vi "add to flattened hierarchy.vi"(8 "error in":errorcluster, 9 "instance data in":T1, 10 "parent ID":string, 11 "flattened hierarchy in":T2) -> (0 "error out":errorcluster, 3 "flattened hierarchy out":T2)   [LabVIEW 2013, in "NISE_CEF_TreeSerializer.lvlib"]
doc: "Add an instance as the child of a given node in the flattened form of the hierarchy"
uses:
  NISE_CEF_TreeSerializer.lvlib
  flat hierarchy.ctl
  full hierarchy.ctl
  hierarchy element.ctl
  instance data.ctl
  NISE_CEF_TreeControl.lvlib
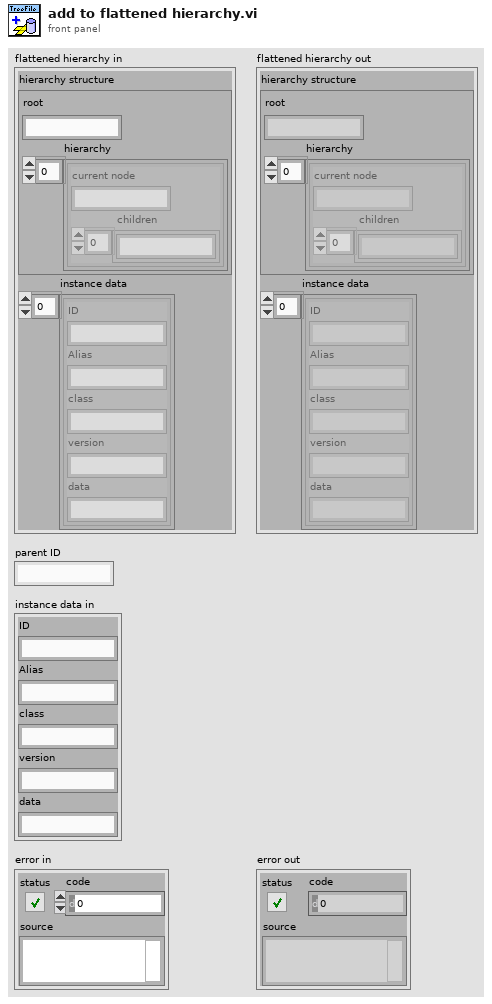
[diagram p1: front panel]
types:
  T1 = typedef "NISE_CEF_TreeSerializer.lvlib/instance data.ctl" = cluster{"ID":string, "Alias":string, "class":string, "version":string, "data":string}
  T2 = typedef "NISE_CEF_TreeSerializer.lvlib/flat hierarchy.ctl" = cluster{"hierarchy structure":T3, "instance data":T1[]}
  T3 = typedef "NISE_CEF_TreeSerializer.lvlib/full hierarchy.ctl" = cluster{"root":string, "hierarchy":T4[]}
  T4 = typedef "NISE_CEF_TreeSerializer.lvlib/hierarchy element.ctl" = cluster{"current node":string, "children":string[]}
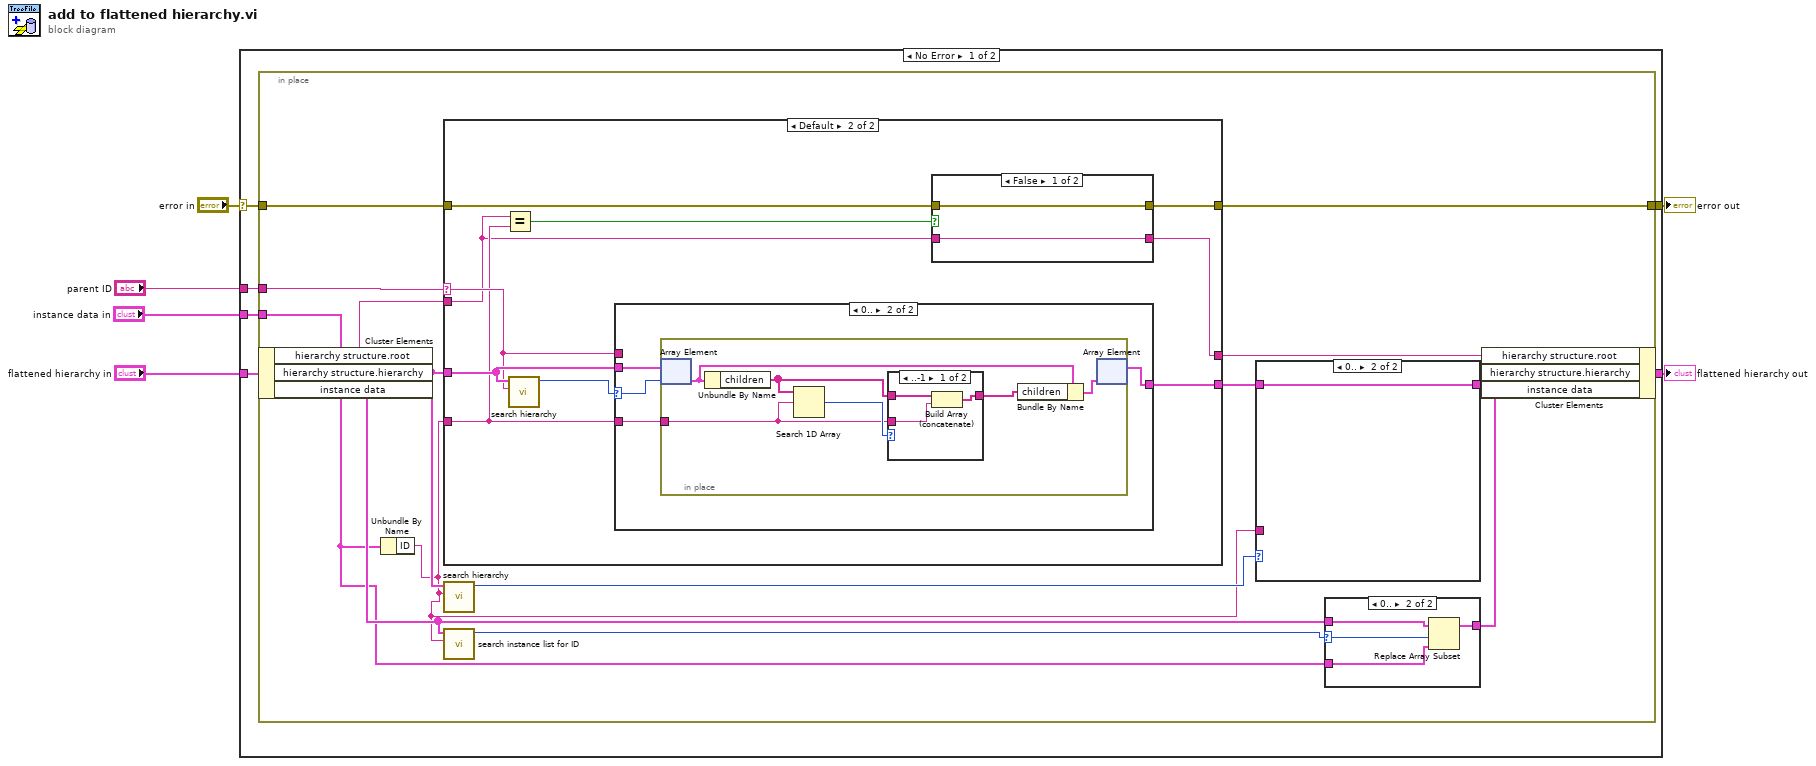
[diagram p0: block diagram]
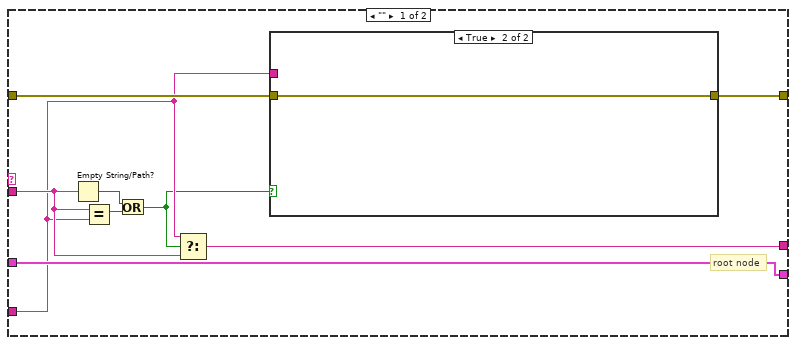
[diagram p2: hidden frame]
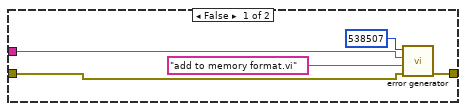
[diagram p3: hidden frame]
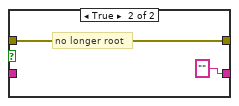
[diagram p4: hidden frame]
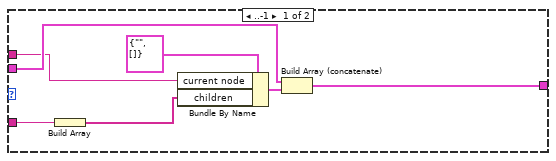
[diagram p5: hidden frame]
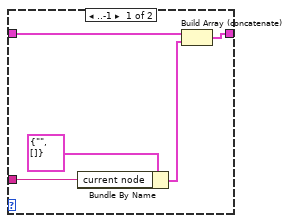
[diagram p7: hidden frame]
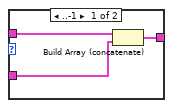
[diagram p8: hidden frame]
diagram:
  n1 = case shown="No Error" "error in" {
    selector: "error in" -> [w8 w91]
    tunnel: [w12 w90] -> w6
    tunnel: "flattened hierarchy in" -> [w11 w90]
    tunnel: "parent ID" -> [w10 _]
    tunnel: "instance data in" -> [w9 _]
    tunnel: [w7 w91] -> w1
    frame No Error {
      n2 = in-place {
        in-place-border: w9 -> [w13]
        in-place-border: w10 -> [w22]
        in-place-border: w8 -> [w17]
        in-place-border: [w16] -> w7
        n3 = in-place-cluster #1(w11) -> ("hierarchy structure.root"=w21:string, "hierarchy structure.hierarchy"=w19:T4[], "instance data"=w25:T1[])
        n4 = Unbundle By Name(w13) -> ("ID"=w14:string)
        n5 = case shown="Default" w22 {
          selector: w22 -> [_ w49]
          tunnel: w19 -> [w35 w50]
          tunnel: [w35 w51] -> w24
          tunnel: w14 -> [w28 w48]
          tunnel: w21 -> [w29 w45]
          tunnel: [w34 w46] -> w20
          tunnel: w17 -> [w33 w43]
          tunnel: [w32 w44] -> w16
          frame "" {
            # "root node"
            n6 = Empty String/Path?(string/path=w29) -> (empty?=w30:bool)
            n7 = Equal?(x=w29, y=w28) -> (x = y?=w31:bool)
            n8 = Or(x=w30, y=w31) -> (x .or. y?=w27:bool)
            n9 = Select(t=w28, s=w27, f=w29) -> (s? t:f=w34:string)
            n10 = case shown="True" w27 {
              tunnel: w33 -> [w40 w41]
              tunnel: [w39 w41] -> w32
              tunnel: w28 -> [w37 _]
              frame False {
                n11 = call "error generator.vi"("error in"=w40, "source"="add to memory format.vi", "append error message"=w37, "error code (0)"=538507) -> ("error out"=w39:errorcluster)  [unwired: 5 in]
              }
              frame True {
              }
            }
          }
          frame Default {
            n12 = Equal?(x=w45, y=w48) -> (x = y?=w47:bool)
            n13 = call "search hierarchy.vi"("ID"=w49, "hierarchy"=w50) -> ("index"=w42:i32)  [unwired: 9 in]
            n14 = case shown="0.." w42 {
              selector: w42 -> [_ w63]
              tunnel: w50 -> [w60 w66]
              tunnel: [w57 w65] -> w51
              tunnel: w48 -> [w59 w64]
              tunnel: w49 -> [w56 _]
              frame ..-1 {
                n15 = Build Array(w59) -> (w58:string[])
                n16 = Bundle By Name(cluster=T4 {"current node"="", "children"=[]} ("hierarchy"), "current node"=w56, "children"=w58) -> (w62:T4)
                n17 = Build Array (concatenate)(w60, w62) -> (w57:T4[])
              }
              frame 0.. {
                n18 = in-place {
                  in-place-border: w64 -> [w68]
                  n19 = in-place-array #2(w66, w63) -> (w72:T4)
                  n20 = Unbundle By Name(w72) -> ("children"=w69:string[])
                  n21 = Search 1D Array(1D array=w69, element=w68) -> (index of element=w70:i32)  [unwired: 1 in]
                  n22 = case shown="..-1" w70 {
                    tunnel: w69 -> [w75 w76]
                    tunnel: w68 -> [w74 _]
                    tunnel: [w73 w76] -> w67
                    frame ..-1 {
                      n23 = Build Array (concatenate)(w75, w74) -> (w73:string[])
                    }
                    frame 0.. {
                    }
                  }
                  n24 = Bundle By Name(cluster=w72, "children"=w67) -> (w71:T4)
                  n25 = in-place-array #2(w71) -> (w65:T4[])  [unwired: 1 out]
                }
              }
            }
            n26 = case shown="False" w47 {
              tunnel: [w53 "" ("root")] -> w46
              tunnel: w45 -> [w53 _]
              tunnel: [w52 w55] -> w44
              tunnel: w43 -> [w52 w55]
              frame False {
              }
              frame True {
                # "no longer root"
              }
            }
          }
        }
        n27 = call "search hierarchy.vi"("ID"=w14, "hierarchy"=w19) -> ("index"=w15:i32)  [unwired: 9 in]
        n28 = call "search instance list for ID.vi"("UID"=w14, "instance data"=w25) -> ("index"=w18:i32)  [unwired: 9 in]
        n29 = case shown="0.." w15 {
          tunnel: w24 -> [w81 w82]
          tunnel: [w80 w82] -> w23
          tunnel: w14 -> [w78 _]
          frame ..-1 {
            n30 = Bundle By Name(cluster=T4 {"current node"="", "children"=[]} ("hierarchy"), "current node"=w78) -> (w77:T4)
            n31 = Build Array (concatenate)(w81, w77) -> (w80:T4[])
          }
          frame 0.. {
          }
        }
        n32 = case shown="0.." w18 {
          selector: w18 -> [_ w86]
          tunnel: [w84 w88] -> w26
          tunnel: w25 -> [w83 w89]
          tunnel: w13 -> [w85 w87]
          frame ..-1 {
            n33 = Build Array (concatenate)(w83, w85) -> (w84:T1[])
          }
          frame 0.. {
            n34 = Replace Array Subset(array=w89, new element=w87, index=w86) -> (w88:T1[])
          }
        }
        n35 = in-place-cluster #1("hierarchy structure.root"=w20, "hierarchy structure.hierarchy"=w23, "instance data"=w26) -> (w12:T2)
      }
    }
    frame Error {
    }
  }
  "flattened hierarchy out" <- w6
  "error out" <- w1
